vi "VISA Send Command.vi"(8 "error in":errorcluster, 10 "Command":string, 11 "34980A in":refnum<class "34980A.lvclass">) -> (0 "error out":errorcluster, 3 "34980A out":refnum<class "34980A.lvclass">)   [LabVIEW 2019, in "34980A.lvlib" / "34980A.lvclass"]
uses:
  Library/34980A.lvclass
  Library/34980A.lvclass/34980A.ctl
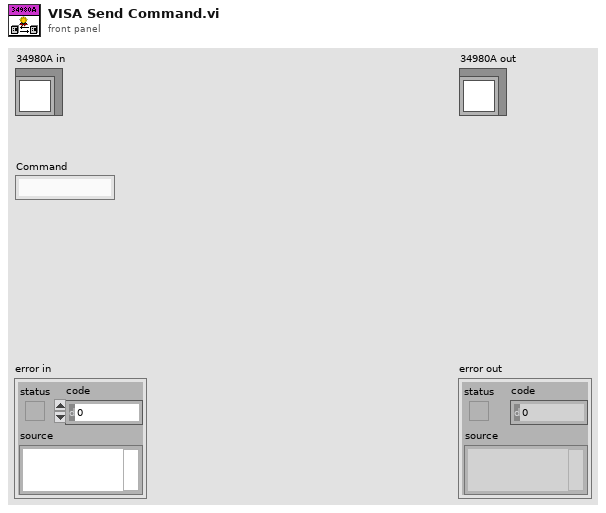
[diagram p1: front panel]
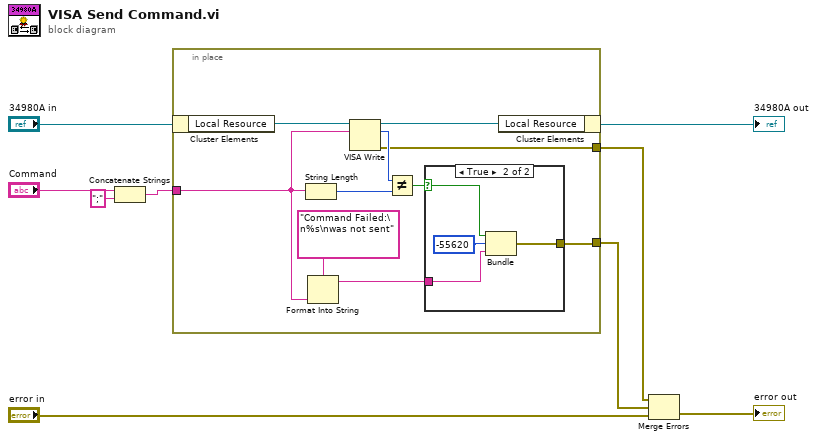
[diagram p0: block diagram]
diagram:
  n1 = Concatenate Strings("Command", ";" ("string")) -> (w2:string)
  n2 = in-place {
    in-place-border: w2 -> [w14]
    in-place-border: [w11] -> w4
    in-place-border: [w10] -> w3
    n3 = in-place-cluster #1("34980A in") -> ("Local Resource"=w19:refnum<visa-resource-name>)
    n4 = String Length(string=w14) -> (length=w17:i32)
    n5 = Format Into String(format string="Command Failed:\n%s\nwas not sent", w14) -> (resulting string=w12:string)  [unwired: 2 in, 1 out]
    n6 = VISA Write(VISA resource name=w19, write buffer=w14) -> (VISA resource name out=w18:refnum<visa-resource-name>, return count=w16:u32, error out=w10:errorcluster)  [unwired: 1 in]
    n7 = Not Equal?(x=w16, y=w17) -> (x != y?=w15:bool)
    n8 = case shown="True" w15 {
      selector: w15 -> [_ w23]
      tunnel: w12 -> [_ w21]
      tunnel: [_ w20] -> w11
      frame False {
      }
      frame True {
        n9 = Bundle(w23, "code"=-55620, w21) -> (w20:cluster{bool, "code":i32, string})  [unwired: 1 in]
      }
    }
    n10 = in-place-cluster #1("Local Resource"=w18) -> (→"34980A out":refnum<class "34980A.lvclass">)
  }
  n11 = Merge Errors(w3, w4, "error in") -> (→"error out":errorcluster)
